vi "Raw data processing-Standard frame data.vi"(11 "Logging queue element":T2 {"Ref Dwell time (us)" format="%#.6g"; "Frame Size" items=["100X100"=100, "128X128"=128, "200X200"=200, "256X256"=256, "512X512"=512, "1024x1024"=1024, "2048x2048"=2048]; "Dwell time (us)" format="%#.6g"}) -> (1 "Single Frame Data":T1, 2 "Number of points in completed standard frame":i32, 3 "Frame completed/generate image":bool)   [LabVIEW 2017]
uses:
  Typedefs/Logging queue element.ctl
  Typedefs/Imaging Protocols enum.ctl
  Typedefs/Frame Size.ctl
  Typedefs/Acquired points count.ctl
  Typedefs/Frame data dual cluster.ctl
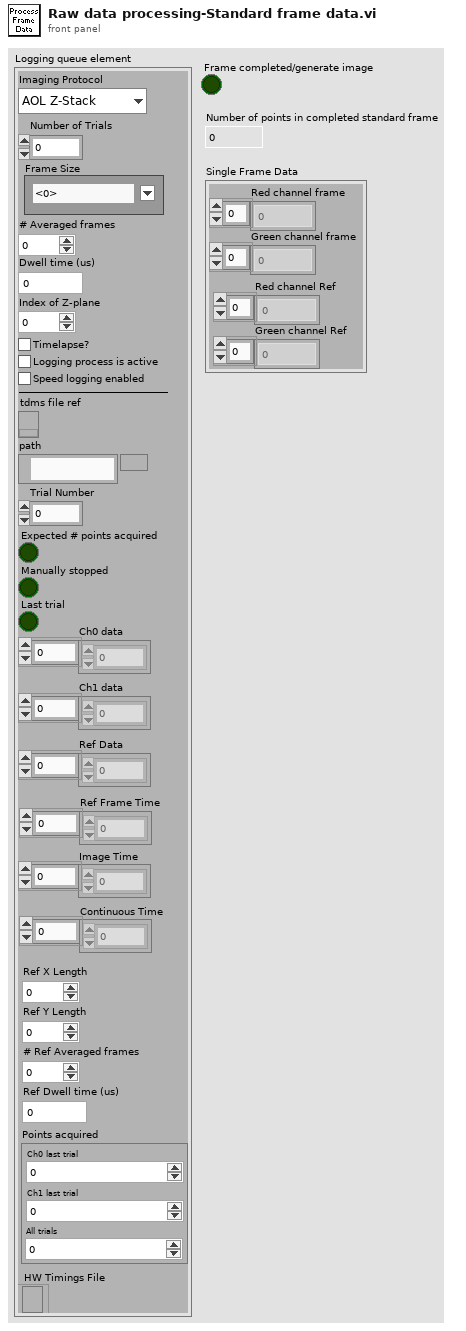
[diagram p1: front panel]
types:
  T1 = typedef "Frame data dual cluster.ctl" = cluster{"Red channel frame":dbl[], "Green channel frame":dbl[], "Red channel Ref":dbl[], "Green channel Ref":dbl[]}
  T2 = typedef "Logging queue element.ctl" = cluster{"Imaging Protocol":T3, "Number of Trials":u16, "Frame Size":T4, "# Averaged frames":u16, "Dwell time (us)":dbl, "Index of Z-plane":i32, "Timelapse?":bool, "Logging process is active":bool, "Speed logging enabled":bool, "tdms file ref":refnum<k34>, "path":path, "Trial Number":i32, "Expected # points acquired":bool, "Manually stopped":bool, "Last trial":bool, "Ch0 data":u32[], "Ch1 data":u32[], "Ref Data":u32[], "Ref Frame Time":u64[], "Image Time":u64[], "Continuous Time":u64[], "Ref X Length":u16, "Ref Y Length":u16, "# Ref Averaged frames":u16, "Ref Dwell time (us)":dbl, "Points acquired":T5, "HW Timings File":refnum<file>}
  T3 = typedef "Imaging Protocols enum.ctl" = enum16{"AOL Z-Stack", "Motor Z Stack", "Functional Acquisition", "Single Plane Acquisition", "Volume Acquisition", "Live Imaging", "Live Plane Imaging", "Live Volume Imaging"}
  T4 = typedef "Frame Size.ctl" = u16
  T5 = typedef "Acquired points count.ctl" = cluster{"Ch0 last trial":u64, "Ch1 last trial":u64, "All trials":u64}
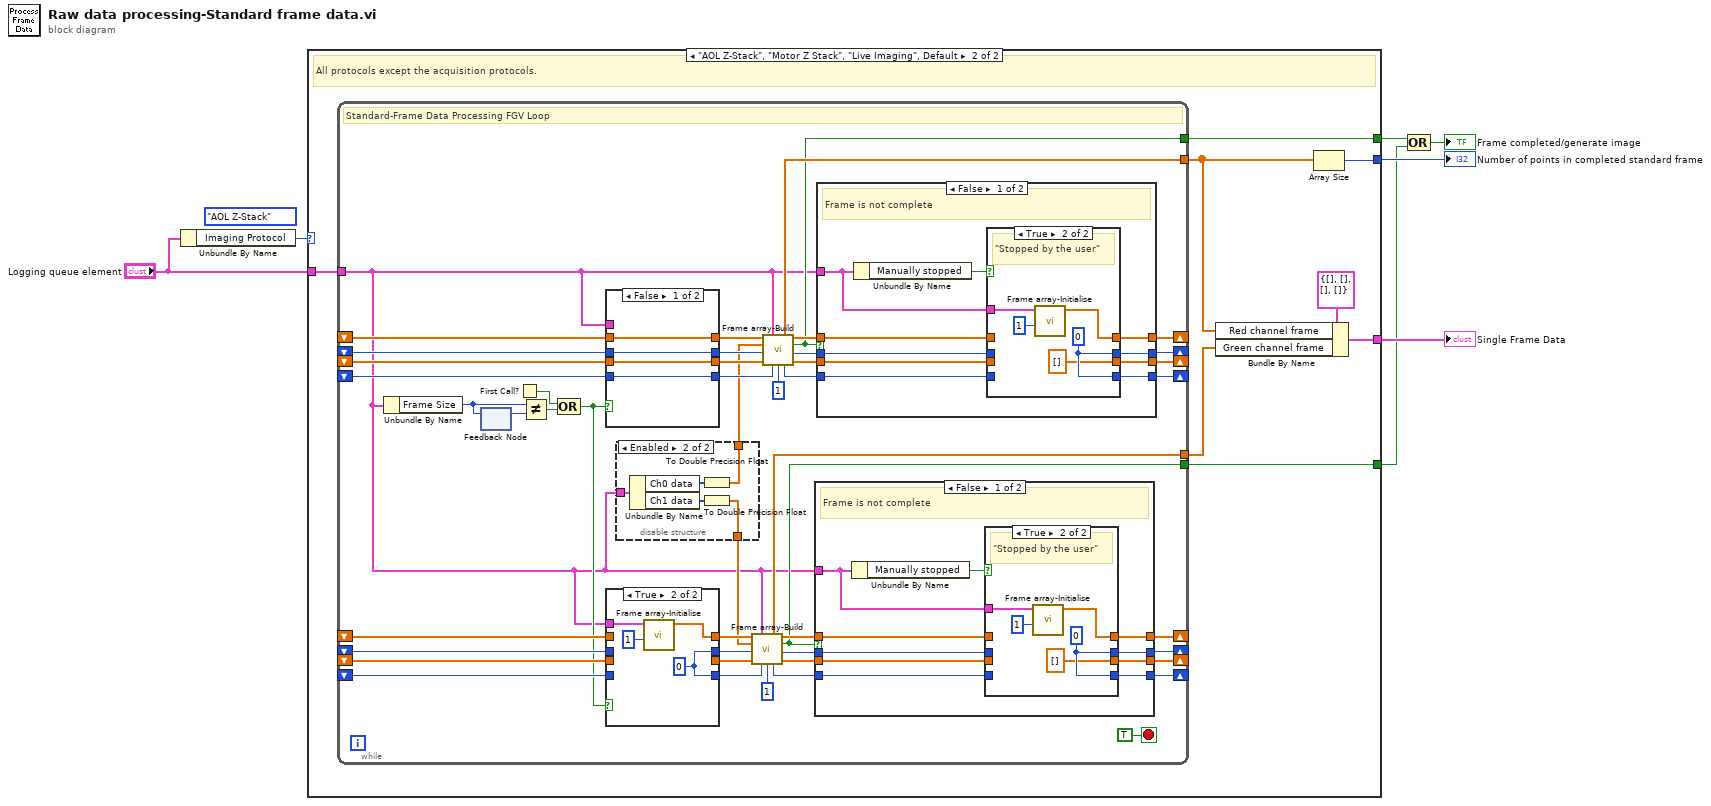
[diagram p0: block diagram]
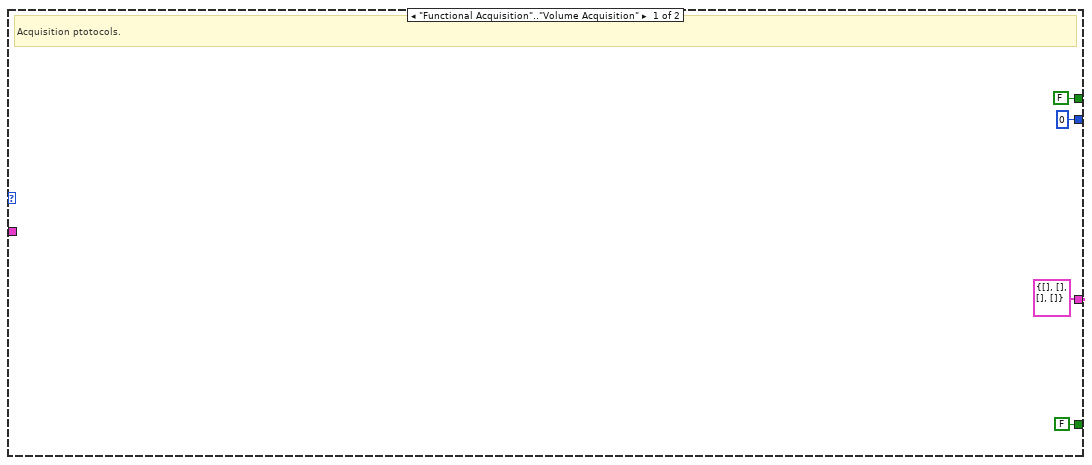
[diagram p2: hidden frame]
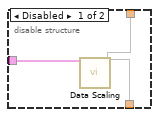
[diagram p3: hidden frame]
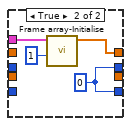
[diagram p7: hidden frame]
diagram:
  (unwired) Imaging_Protocols_enum."AOL Z-Stack" ("Imaging Protocol")
  n1 = Unbundle By Name("Logging queue element") -> ("Imaging Protocol"=w5:T3)
  n2 = case shown="\"AOL Z-Stack\", \"Motor Z Stack\", \"Live Imaging\", Default" w5 {
    tunnel: "Logging queue element" -> [_ w19]
    tunnel: [FALSE ("Frame completed/generate image") w18] -> w2
    tunnel: [T1 {"Red channel frame"=[], "Green channel frame"=[], "Red channel Ref"=[], "Green channel Ref"=[]} ("Single Frame Data") w15] -> w6
    tunnel: [0 w14] -> w7
    tunnel: [FALSE ("Frame completed/generate image") w12] -> w1
    frame "Functional Acquisition".."Volume Acquisition" {
      # "Acquisition ptotocols."
    }
    frame "AOL Z-Stack", "Motor Z Stack", "Live Imaging", Default {
      # "All protocols except the acquisition protocols."
      n3 = while {
        tunnel: w19 -> [w20]
        shift-right: [w65] -> _
        shift-left: _ -> [w61]
        shift-right: [w60] -> _
        shift-left: _ -> [w59]
        shift-right: [w50] -> _
        shift-left: _ -> [w52]
        shift-right: [w49] -> _
        shift-left: _ -> [w48]
        tunnel: [w45] -> w13
        tunnel: [w42] -> w18
        shift-right: [w25] -> _
        shift-left: _ -> [w26]
        shift-right: [w27] -> _
        shift-left: _ -> [w28]
        shift-right: [w36] -> _
        shift-left: _ -> [w34]
        shift-right: [w37] -> _
        shift-left: _ -> [w38]
        tunnel: [w24] -> w16
        tunnel: [w23] -> w12
        stop <- TRUE stop-if-true
        # "Standard-Frame Data Processing FGV Loop"
        n4 = Unbundle By Name(w20) -> ("Frame Size"=w55:T4)
        n5 = feedback #1() -> (w62:T4)  [unwired: 1 in]
        n6 = feedback-in #1(w55) -> ()
        n7 = First Call?() -> (First Call?: T/F=w64:bool)
        n8 = Not Equal?(x=w55, y=w62) -> (x != y?=w63:bool)
        n9 = Compound Arithmetic op=OR(w64, w63) -> (w21:bool)
        n10 = case shown="False" w21 {
          tunnel: [w109 w112] -> w54
          tunnel: w61 -> [w109 _]
          tunnel: w20 -> [_ w113]
          tunnel: w59 -> [w108 _]
          tunnel: [w108 w110] -> w58
          tunnel: [w107 _] -> w53
          tunnel: w52 -> [w107 _]
          tunnel: w48 -> [w106 _]
          tunnel: [w106 w110] -> w47
          frame False {
          }
          frame True {
            w110 = 0 ("Count")
            n11 = call "Frame array-Initialise.vi"("Number of channels in array"=1, "Logging queue element"=w113) -> ("Frame-size data array (single channel)"=w112:dbl[])  [unwired: 9 in]
          }
        }
        n12 = case shown="True" w21 {
          tunnel: [w78 w81] -> w32
          tunnel: w26 -> [w78 _]
          tunnel: w20 -> [_ w82]
          tunnel: w28 -> [w77 _]
          tunnel: [w77 w79] -> w29
          tunnel: [w76 _] -> w33
          tunnel: w34 -> [w76 _]
          tunnel: w38 -> [w75 _]
          tunnel: [w75 w79] -> w39
          frame False {
          }
          frame True {
            w79 = 0 ("Count")
            n13 = call "Frame array-Initialise.vi"("Number of channels in array"=1, "Logging queue element"=w82) -> ("Frame-size data array (single channel)"=w81:dbl[])  [unwired: 9 in]
          }
        }
        n14 = disable-structure shown="Enabled" {
          disable-tunnel: [w69 w72] -> w44
          disable-tunnel: [w68 w70] -> w22
          disable-tunnel: w20 -> [w67 w74]
          frame Disabled {
            n15 = call "Data Scaling.vi"("Logging queue element in"=w67) -> (4:w69, 6:w68)  [unwired: 11 in, 2 out]
          }
          frame Enabled {
            n16 = Unbundle By Name(w74) -> ("Ch0 data"=w73:u32[], "Ch1 data"=w71:u32[])
            n17 = To Double Precision Float(number=w73) -> (double precision float=w72:dbl[])
            n18 = To Double Precision Float(number=w71) -> (double precision float=w70:dbl[])
          }
        }
        n19 = call "Frame array-Build.vi"("Single-frame buffer (in)"=w32, "Logging queue element"=w20, "New chunk of scaled data (single channel)"=w22, "Number of points in single-frame buffer (in)"=w29, "Frame values sum (in)"=w33, "Averaged frames count (in)"=w39, "Number of channels in input data array"=1) -> ("Frame Data"=w24:dbl[], "Single-frame buffer (out)"=w30:dbl[], "Frame completed/generate image"=w23:bool, "Number of points in single-frame buffer (out)"=w31:i32, "Averaged frames count (out)"=w40:i32, "Frame values sum (out)"=w35:dbl[])  [unwired: 3 in]
        n20 = call "Frame array-Build.vi"("Single-frame buffer (in)"=w54, "Logging queue element"=w20, "New chunk of scaled data (single channel)"=w44, "Number of points in single-frame buffer (in)"=w58, "Frame values sum (in)"=w53, "Averaged frames count (in)"=w47, "Number of channels in input data array"=1) -> ("Frame Data"=w45:dbl[], "Single-frame buffer (out)"=w57:dbl[], "Frame completed/generate image"=w42:bool, "Number of points in single-frame buffer (out)"=w56:i32, "Averaged frames count (out)"=w46:i32, "Frame values sum (out)"=w51:dbl[])  [unwired: 3 in]
        n21 = case shown="False" w23 {
          tunnel: w30 -> [w90 w105]
          tunnel: [w92 w105] -> w25
          tunnel: w31 -> [w88 w103]
          tunnel: [w87 w103] -> w27
          tunnel: w20 -> [w89 _]
          tunnel: w35 -> [w86 w104]
          tunnel: [w85 w104] -> w36
          tunnel: w40 -> [w84 w102]
          tunnel: [w83 w102] -> w37
          frame False {
            # "Frame is not complete"
            n22 = Unbundle By Name(w89) -> ("Manually stopped"=w91:bool)
            n23 = case shown="True" w91 {
              tunnel: [w96 w101] -> w92
              tunnel: w90 -> [w96 _]
              tunnel: w89 -> [_ w100]
              tunnel: w88 -> [w95 _]
              tunnel: [w95 w99] -> w87
              tunnel: w86 -> [w94 _]
              tunnel: [w94 dbl[] [] ("Frame-size data array out")] -> w85
              tunnel: w84 -> [w93 _]
              tunnel: [w93 w99] -> w83
              frame False {
                # "Not stopped"
              }
              frame True {
                w99 = 0 ("Count")
                # "\"Stopped by the user\""
                n24 = call "Frame array-Initialise.vi"("Number of channels in array"=1, "Logging queue element"=w100) -> ("Frame-size data array (single channel)"=w101:dbl[])  [unwired: 9 in]
              }
            }
          }
          frame True {
            # "Frame completed (or Av. frame completed if averaging)"
          }
        }
        n25 = case shown="False" w42 {
          tunnel: w57 -> [w121 w136]
          tunnel: [w123 w136] -> w65
          tunnel: w56 -> [w119 w134]
          tunnel: [w118 w134] -> w60
          tunnel: w20 -> [w120 _]
          tunnel: w51 -> [w117 w135]
          tunnel: [w116 w135] -> w50
          tunnel: w46 -> [w115 w133]
          tunnel: [w114 w133] -> w49
          frame False {
            # "Frame is not complete"
            n26 = Unbundle By Name(w120) -> ("Manually stopped"=w122:bool)
            n27 = case shown="True" w122 {
              tunnel: [w127 w132] -> w123
              tunnel: w121 -> [w127 _]
              tunnel: w120 -> [_ w131]
              tunnel: w119 -> [w126 _]
              tunnel: [w126 w130] -> w118
              tunnel: w117 -> [w125 _]
              tunnel: [w125 dbl[] [] ("Frame-size data array out")] -> w116
              tunnel: w115 -> [w124 _]
              tunnel: [w124 w130] -> w114
              frame False {
                # "Not stopped"
              }
              frame True {
                w130 = 0 ("Count")
                # "\"Stopped by the user\""
                n28 = call "Frame array-Initialise.vi"("Number of channels in array"=1, "Logging queue element"=w131) -> ("Frame-size data array (single channel)"=w132:dbl[])  [unwired: 9 in]
              }
            }
          }
          frame True {
            # "Frame completed (or Av. frame completed if averaging)"
          }
        }
      }
      n29 = Bundle By Name(cluster=T1 {"Red channel frame"=[], "Green channel frame"=[], "Red channel Ref"=[], "Green channel Ref"=[]} ("Single Frame Data"), "Red channel frame"=w13, "Green channel frame"=w16) -> (w15:T1)
      n30 = Array Size(array=w13) -> (size(s)=w14:i32)
    }
  }
  "Number of points in completed standard frame" <- w7
  "Single Frame Data" <- w6
  n31 = Compound Arithmetic op=OR(w2, w1) -> (→"Frame completed/generate image":bool)
